vi "Diagram Get Execution Order debug.vi"(8 "Error In":errorcluster) -> (0 "Error Out":errorcluster)   [LabVIEW 2018]
panel:
  out "Array 2":string[](array[string])
  out "Class Hierarchy":string[][](array[string])
  in  "vi path":path=path "C:/Users/lubo/Documents/LabView/LabVIEW-Universal-Transcriptor/Test/Examples For Parsing/Blink 2.vi"
  out "Array":string[](array[string])
  in  "Diag Refnum":refnum<vi>
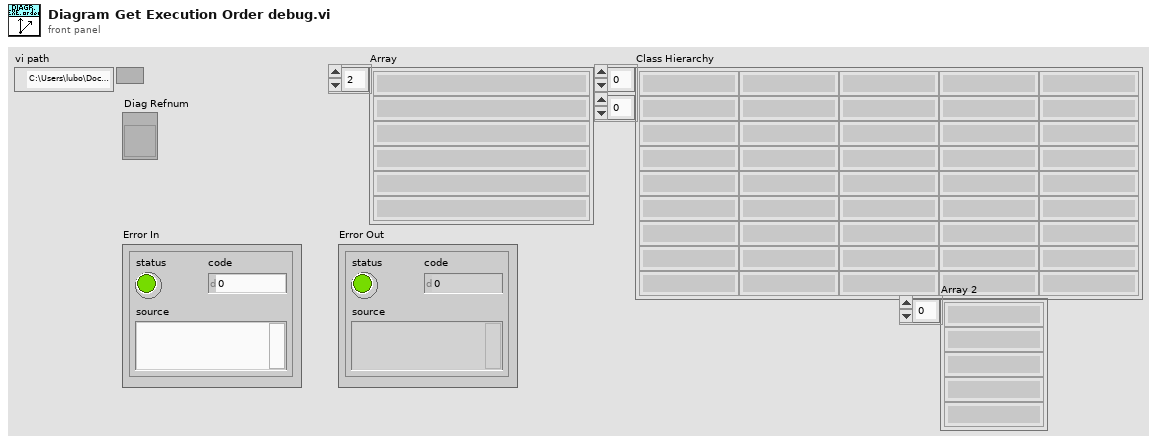
[diagram p1: front panel]
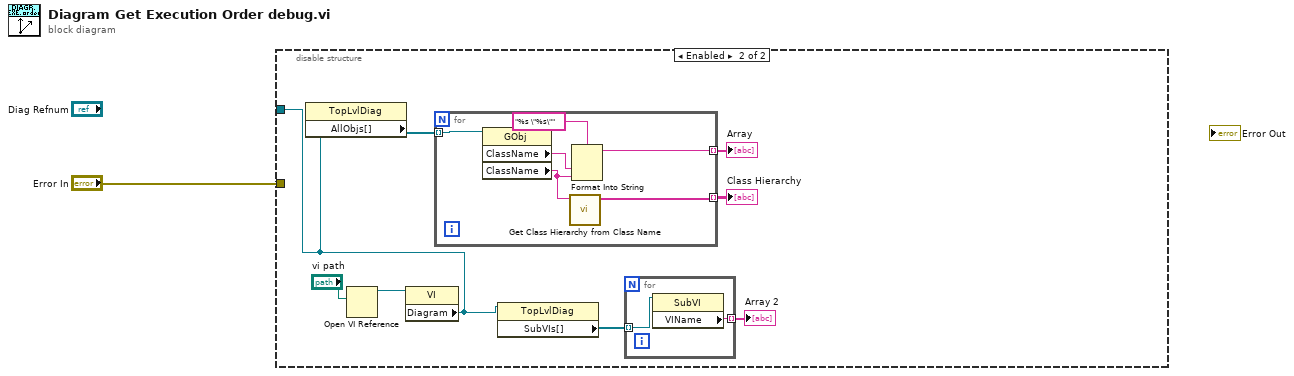
[diagram p0: block diagram]
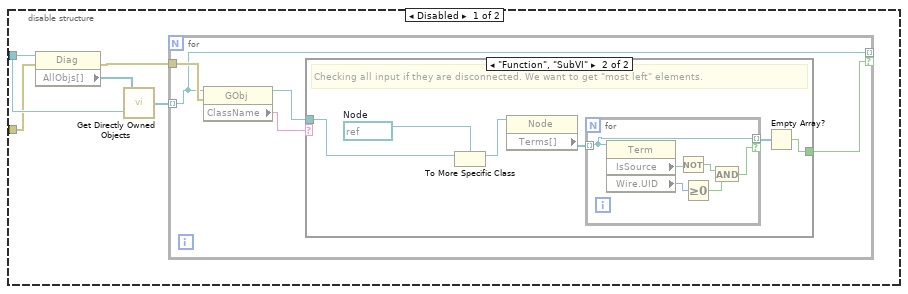
[diagram p2: hidden frame]
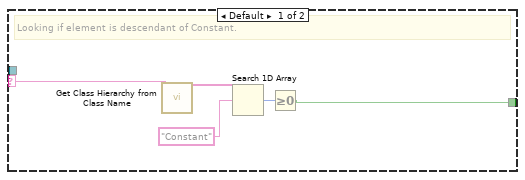
[diagram p3: hidden frame]
diagram:
  n1 = disable-structure shown="Enabled" {
    disable-tunnel: [w6 w31] -> _
    disable-tunnel: "Error In" -> [w4 _]
    frame Disabled {
      n2 = property class="Diag"(reference=w6, error in=w4) -> (error out=w2:errorcluster, "AllObjs[]"=w5:refnum<vi>[])  [unwired: 1 out]
      n3 = call "Get Directly Owned Objects.vi"("Top Object"=w6, "Nested Objects"=w5) -> ("Directly Owned Objects"=w3:refnum<vi>[])
      n4 = for {
        tunnel: w3 -> [w10] mode=indexing
        tunnel: w2 -> [w11]
        tunnel: [w10] -> _ mode=indexing if=w8
        n5 = property class="GObj"(reference=w10, error in=w11) -> (reference out=w7:refnum<vi>, "ClassName"=w9:string)  [unwired: 1 out]
        n6 = case shown="\"Function\", \"SubVI\"" w9 {
          selector: w9 -> [w16 _]
          tunnel: [w12 w17] -> w8
          tunnel: w7 -> [_ w22]
          frame Default {
            # "Looking if element is descendant of Constant."
            n7 = call <vilib>:"Get Class Hierarchy from Class Name.vi"("Class Name"=w16) -> ("Class Hierarchy"=w15:string[])  [unwired: 9 in, 1 out]
            n8 = Search 1D Array(1D array=w15, element="Constant") -> (index of element=w13:i32)  [unwired: 1 in]
            n9 = Greater Or Equal To 0?(x=w13) -> (x >= 0?=w12:bool)
          }
          frame "Function", "SubVI" {
            w21 = refnum<vi> refnum  # Node
            # "Checking all input if they are disconnected. We want to get \"most left\" elements."
            n10 = To More Specific Class(target class=w21, reference=w22) -> (specific class reference=w20:refnum<vi>)  [unwired: 1 in, 1 out]
            n11 = property class="Node"(reference=w20) -> ("Terms[]"=w19:refnum<vi>[])  [unwired: 1 in, 2 out]
            n12 = for {
              tunnel: w19 -> [w24] mode=indexing
              tunnel: [w24] -> w18 mode=indexing if=w23
              n13 = property class="Term"(reference=w24) -> ("IsSource"=w28:bool, "Wire.UID"=w27:i32)  [unwired: 1 in, 2 out]
              n14 = Not(x=w28) -> (.not. x?=w26:bool)
              n15 = Greater Or Equal To 0?(x=w27) -> (x >= 0?=w25:bool)
              n16 = And(x=w26, y=w25) -> (x .and. y?=w23:bool)
            }
            n17 = Empty Array?(array=w18) -> (empty?=w17:bool)
          }
        }
      }
    }
    frame Enabled {
      n18 = Open VI Reference(vi path="vi path") -> (vi reference=w33:refnum<vi>)  [unwired: 5 in, 1 out]
      n19 = property class="VI"(reference=w33) -> ("Diagram"=w31:refnum<vi>)  [unwired: 1 in, 2 out]
      n20 = property class="TopLvlDiag"(reference=w31) -> ("AllObjs[]"=w36:refnum<vi>[])  [unwired: 1 in, 2 out]
      n21 = for {
        tunnel: w36 -> [w44] mode=indexing
        tunnel: [w41] -> w35 mode=indexing
        tunnel: [w39] -> w32 mode=indexing
        n22 = property class="GObj"(reference=w44) -> ("ClassName"=w43:string, "ClassName"=w40:string)  [unwired: 1 in, 2 out]
        n23 = call <vilib>:"Get Class Hierarchy from Class Name.vi"("Class Name"=w40) -> ("Class Hierarchy"=w39:string[])  [unwired: 9 in, 1 out]
        n24 = Format Into String(format string="%s \"%s\"", w43, w40) -> (resulting string=w41:string)  [unwired: 2 in, 1 out]
      }
      "Array" <- w35
      "Class Hierarchy" <- w32
      n25 = property class="TopLvlDiag"(reference=w31) -> ("SubVIs[]"=w30:refnum<vi>[])  [unwired: 1 in, 2 out]
      n26 = for {
        tunnel: w30 -> [w38] mode=indexing
        tunnel: [w37] -> w29 mode=indexing
        n27 = property class="SubVI"(reference=w38) -> ("VIName"=w37:string)  [unwired: 1 in, 2 out]
      }
      "Array 2" <- w29
    }
  }
